vi "Read Data.vi"(8 "error in (no error)":errorcluster caption="错误输入（无错误）", 11 "EPEVER-MPPT 输入":refnum<class "EPEVER-MPPT.lvclass">) -> (0 "error out":errorcluster caption="错误输出", 3 "EPEVER-MPPT 输出":refnum<class "EPEVER-MPPT.lvclass">)   [LabVIEW 2016, in "EPEVER-MPPT.lvlib" / "EPEVER-MPPT.lvclass"]
uses:
  EPEVER-MPPT.lvclass
  EPEVER-MPPT.lvclass/EPEVER-MPPT.ctl
  <vilib>/Plasmionique/MB Master/MB Master.lvlib
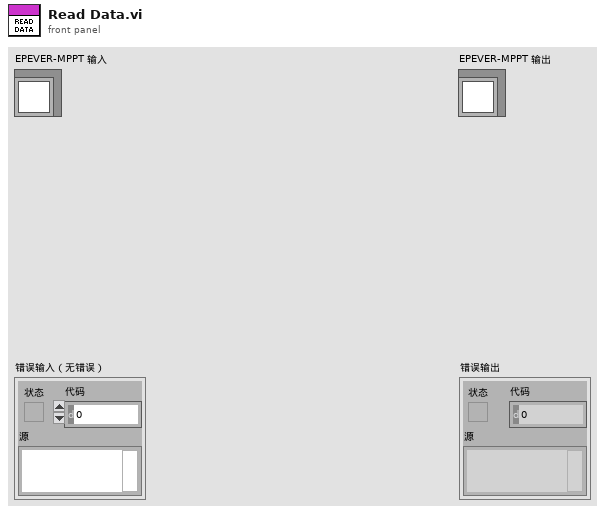
[diagram p1: front panel]
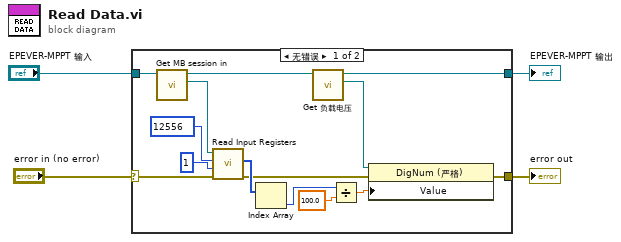
[diagram p0: block diagram]
diagram:
  n1 = case shown="无错误" "error in (no error)" {
    selector: "error in (no error)" -> [w14 w20]
    tunnel: [w5 w20] -> w3
    tunnel: [w7 w19] -> w1
    tunnel: "EPEVER-MPPT 输入" -> [w18 w19]
    frame No Error {
      n2 = call "Get MB session in.vi"("EPEVER-MPPT in"=w18) -> ("MB Serial Master:MB_Master"=w17:refnum<class "MB_Master.lvclass">, "EPEVER-MPPT out"=w13:refnum<class "EPEVER-MPPT.lvclass">)  [unwired: 9 in]
      n3 = call <vilib>:"Read Input Registers.vi"("error in (no error)"=w14, "quantity"=u16 1, "starting address"=u16 12556, "MB session in"=w17) -> ("error out"=w6:errorcluster, "Registers"=w11:u16[])  [unwired: 5 in, 1 out]
      n4 = Index Array(array=w11) -> (element=w10:u16)  [unwired: 1 in]
      n5 = call "Get 负载电压.vi"("EPEVER-MPPT in"=w13) -> ("负载电压"=w12:refnum<vi>, "EPEVER-MPPT out"=w7:refnum<class "EPEVER-MPPT.lvclass">)  [unwired: 9 in]
      n6 = Divide(x=w10, y=100.0) -> (x/y=w8:dbl)
      n7 = property class="DigNum (严格)"(reference=w12, error in=w6, "Value"=w8) -> (error out=w5:errorcluster)  [unwired: 1 out]
    }
    frame Error {
    }
  }
  "error out" <- w3
  "EPEVER-MPPT 输出" <- w1
